vi "deco_ee_492.vi"(5 "mapaeeprom":string) -> (0 "Med_caract":string, 1 "Med_unid":string[](array[string]), 2 "Med_nom":string[](array[string]), 3 "cantmedic":u8)   [LabVIEW 2010]
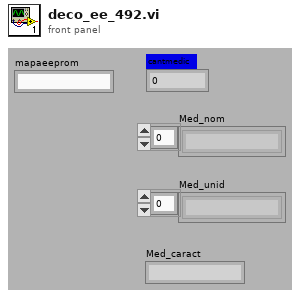
[diagram p1: front panel]
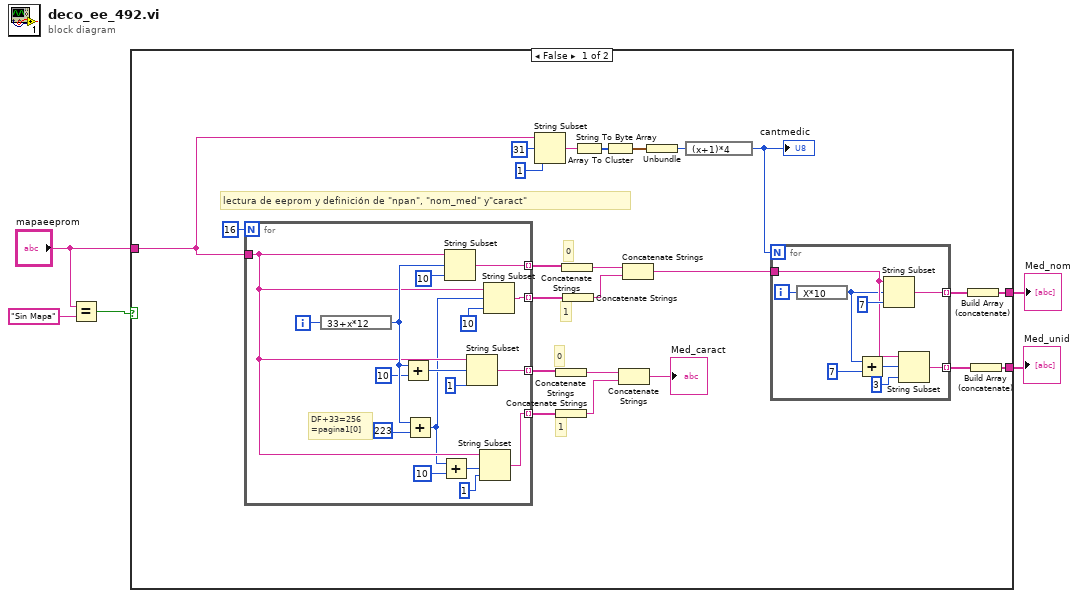
[diagram p0: block diagram]
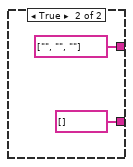
[diagram p2: hidden frame]
diagram:
  n1 = Equal?(x="mapaeeprom", y="Sin Mapa") -> (x = y?=w1:bool)
  n2 = case shown="False" w1 {
    tunnel: [w16 string[] []] -> w5
    tunnel: [w9 string[] ["", "", ""]] -> w4
    tunnel: "mapaeeprom" -> [w6 _]
    frame False {
      # "lectura de eeprom y definición de \"npan\", \"nom_med\" y\"caract\""
      # "1"
      # "0"
      # "1"
      # "0"
      n3 = for {
        N: 16 -> [_]
        tunnel: w6 -> [w45]
        tunnel: [w50] -> w18 mode=indexing
        tunnel: [w49] -> w19 mode=indexing
        tunnel: [w40] -> w20 mode=indexing
        tunnel: [w39] -> w21 mode=indexing
        i -> [w53]
        # "DF+33=256\n=pagina1[0]"
        n4 = expression code="33+x*12"(w53) -> (w47:i32)
        n5 = Add(x=w47, y=u8 10) -> (x+y=w46:i32)
        n6 = Add(x=w47, y=u8 223) -> (x+y=w43:i32)
        n7 = Add(x=w43, y=10) -> (x+y=w41:i32)
        n8 = String Subset(string=w45, offset (0)=w47, length (rest)=10 ("length (rest)")) -> (substring=w50:string)
        n9 = String Subset(string=w45, offset (0)=w46, length (rest)=1 ("length (rest)")) -> (substring=w39:string)
        n10 = String Subset(string=w45, offset (0)=w41, length (rest)=1 ("length (rest)")) -> (substring=w40:string)
        n11 = String Subset(string=w45, offset (0)=w43, length (rest)=10 ("length (rest)")) -> (substring=w49:string)
      }
      n12 = String Subset(string=w6, offset (0)=31, length (rest)=1 ("length (rest)")) -> (substring=w8:string)
      n13 = Concatenate Strings(w21) -> (w24:string)
      n14 = Concatenate Strings(w20) -> (w25:string)
      n15 = Concatenate Strings(w18) -> (w22:string)
      n16 = Concatenate Strings(w19) -> (w23:string)
      n17 = String To Byte Array(string=w8) -> (unsigned byte array=w12:u8[])
      n18 = Array To Cluster(array=w12) -> (cluster=w11:cluster{"unsigned byte array[0]":u8})
      n19 = Concatenate Strings(w24, w25) -> (→"Med_caract":string)
      n20 = Concatenate Strings(w22, w23) -> (w7:string)
      n21 = Unbundle(w11) -> ("unsigned byte array[0]"=w13:u8)
      n22 = expression code="(x+1)*4"(w13) -> (w10:u8)
      "cantmedic" <- w10
      n23 = for {
        N: w10 -> [_]
        tunnel: w7 -> [w32]
        tunnel: [w35] -> w15 mode=indexing
        tunnel: [w31] -> w14 mode=indexing
        i -> [w36]
        n24 = expression code="X*10"(w36) -> (w30:i32)
        n25 = Add(x=w30, y=7 ("x")) -> (x+y=w33:i32)
        n26 = String Subset(string=w32, offset (0)=w30, length (rest)=7 ("length (rest)")) -> (substring=w35:string)
        n27 = String Subset(string=w32, offset (0)=w33, length (rest)=3 ("length (rest)")) -> (substring=w31:string)
      }
      n28 = Build Array (concatenate)(w15) -> (w9:string[])
      n29 = Build Array (concatenate)(w14) -> (w16:string[])
    }
    frame True {
    }
  }
  "Med_unid" <- w5
  "Med_nom" <- w4
